vi "Avs47Ave.vi"() -> ()   [LabVIEW 2012]
doc: "Application example"
uses:
  <vilib>/ptbypt/NI_PtbyPt.lvlib
panel:
  out "VISA RESOURCE":refnum<visa-resource-name>
  in  "FIXED/AUTOSCALE":bool=TRUE
  out "AUTOSCALE CHART":i32(graph)
  in  "OFFSET/SCALE ADJ.":bool=TRUE
  out "AL ERROR":bool
  out "PEAK-TO-PEAK":dbl format="%_3f"
  out "LAST READING  AS STRING":string="000.000 ohm"
  out "PP/STD RATIO":dbl format="%.1f"
  out "READING No.":i32=1
  out "turns":i32
  in  "SAMPLE LENGTH":i32=300
  in  "RE-START MEASUREMENT":bool
  out "AVERAGE":dbl format="%^_5e"
  out "STD":dbl format="%_3f"
  out "FIXED SCALE CHART":i32(graph)
  out "LABVIEW ERROR":errorcluster
  out "OVERRANGE":bool
  out "ADC READING":i32
  in  "stop":bool
  in  "DIGITAL REFERENCE":u16 max=20475 step=1
  in  "DISPLAY":u8(ring) items=["530A SET PT"=7, "530A HEAT I"=6, "530A HEAT V"=5, "EXC VOLT"=4, "REFERENCE"=3, "ADJ REF"=2, "DR"=1, "R"=0]
  in  "EXCITATION":u8(ring)=7 items=["3mV"=7, "1mV"=6, "300uV"=5, "100uV"=4, "30uV"=3, "10uV"=2, "3 uV"=1, "NO EXCITATION"=0]
  in  "RANGE":u8(ring)=3 items=["2 MOhms"=7, "200 kOhms"=6, "20 kOhms"=5, "2 kOhms"=4, "200 Ohms"=3, "20 Ohms"=2, "2 Ohms"=1, "NO RANGE"=0]
  in  "CHANNEL":u8(ring) items=["CH7"=7, "CH6"=6, "CH5"=5, "CH4"=4, "CH3"=3, "CH2"=2, "CH1"=1, "CH0"=0]
  in  "INPUT":u8(ring)=2 items=["CAL"=2, "MEAS"=1, "ZERO"=0]
  in  "REMOTE":u8(ring) items=["YES"=1, "NO"=0]
  # "AVS47AVE.VI  NOISE AND CALIBRATION TEST PROGRAM FOR AVS-47B"
  # "RV-ELEKTRONIIKKA OY\nPICOWATT"
  # "The following port has been opened for the\nVISA session."
  # "NOTE 1:  Following settings must be made before starting the program: Sample length, Manual/Autoscale, Offset/Scale adj.\nNOTE 2:  Check the port that your computer is using as the VISA resource for the USB-232 converter.  Load, modify and run \n                 \"CreateDefaultConfigurationCluster.vi\" if it indicated an incorrect VISA resource."
  # "This VI can be used for testing the AVS-47B both in remote and local modes. The main use is testing noise and adjusting scale factor for the seven\nexcitation ranges. The bridge configuration can be changed after the program has started. Recording data can be re-started when\nrunning. \n\n- LAST READING is the AVS-47B display,  shown as a string with resistance unit appended for convenient reading.\n- AVERAGE is the mean value of [sample length] readings in ohms. If sample length has not yet been reached, AVERAGE  is the mean of \n   readings taken so far.\n- STD is the standard deviation of [sample length] readings in ohms. If sample length has not yet been reached, STD is the standard deviation\n   of readings taken so far.\n- PP/STD ratio should be about 5 for random noise and a large number of samples. A number much less than 5 is probably due to\n  too few readings. A number much higher than 5 is probably due to external interference (spikes), or too few samples.  On high excitation\n   ranges, digital steps can produce too low or too high PP/STD ratios.\n- ADC reading should be viewed if the DISPLAY is not R or 1xdR.  Calibration of excitation ranges should be done  at middle scale \n(reading 10000). \n- OVERRANGE indicator is set, if the voltage entering the A/D converter exceeds 1.9999 Volts (the ADC reading is  0 during overload)\n- AL ERROR tells that syncronisation to the ADC fails because the AL signal never comes true. This can happen if a wrong port was \n   opened as the  VISA resource, or if the  connection between AVS-47B and the computer fails.\n- If FIXED SCALE is selected, choose either OFFSET OR SCALE for \"OFFSET/SCALE ADJ\".  This centers the scale around 0 or 10000. The\n   low and high limits of the amplitude axis are automatically determined on the basis of the selected excitation range."
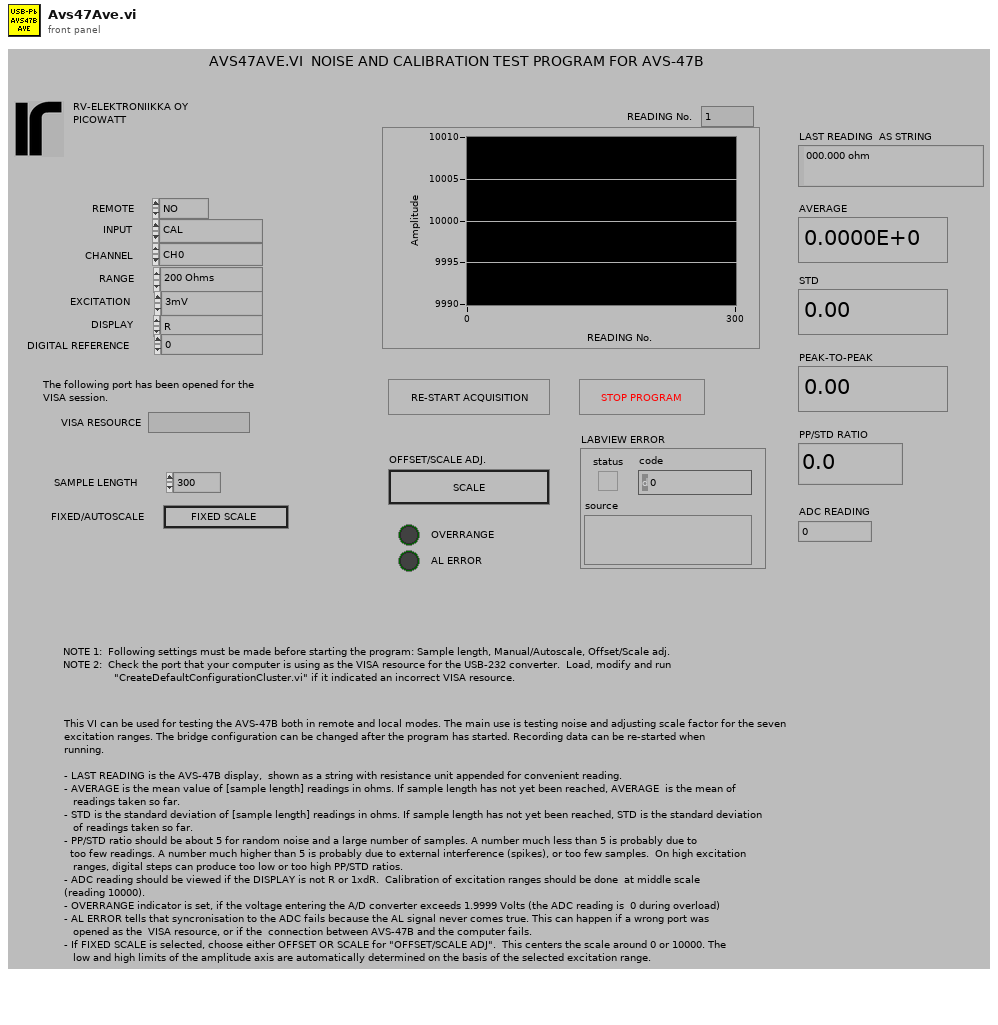
[diagram p1: front panel]
types:
  T1 = cluster{"VISA RESOURCE":refnum<visa-resource-name>, "PICOBUS ADDRESS":u8, "DISABLE AL":u8, "REMOTE":u8, "INPUT":u8, "CHANNEL":u8, "RANGE":u8, "EXCITATION":u8, "DISPLAY":u8, "DIGITAL REFERENCE":u16, "SET POINT":dbl, "PROP GAIN":u8, "INTG":u8, "DERIV":u8, "POWER BIAS":u8, "POWER RANGE":u8, "INFO STRING":string, "HEATER RESISTANCE":dbl, "INTERVAL":u8, " SENSOR dR/dT":u8}
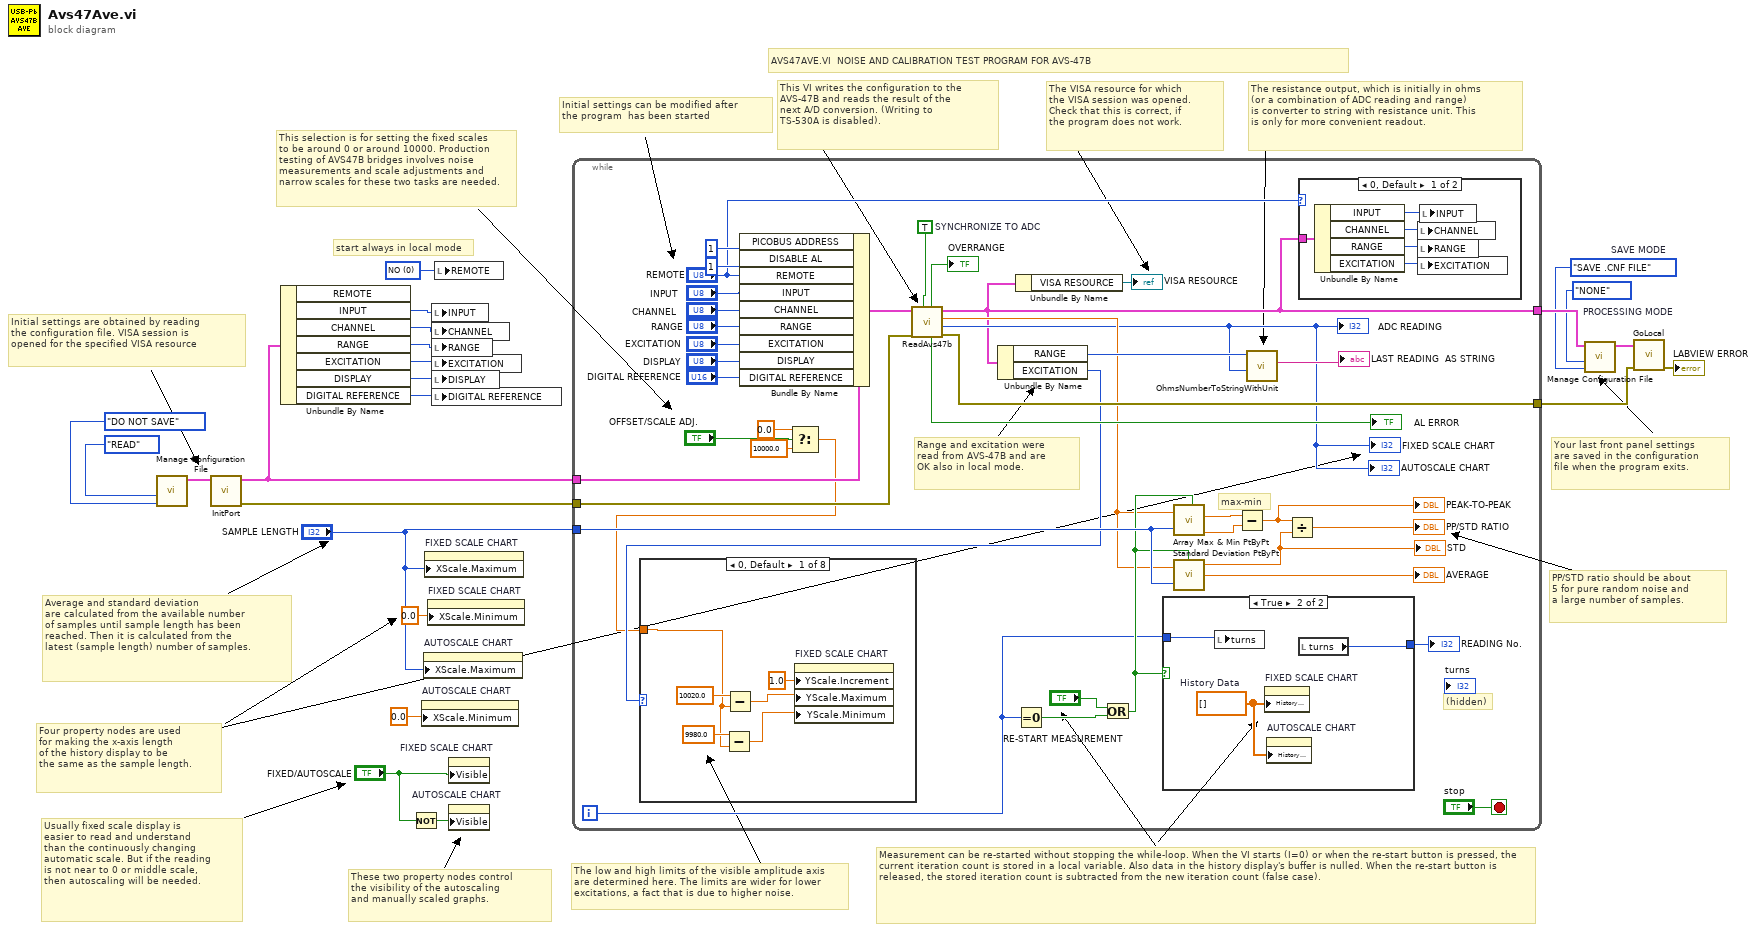
[diagram p0: block diagram]
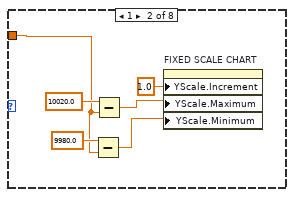
[diagram p3: hidden frame]
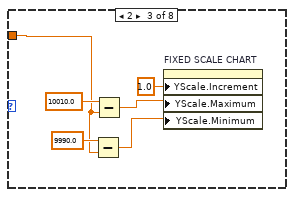
[diagram p4: hidden frame]
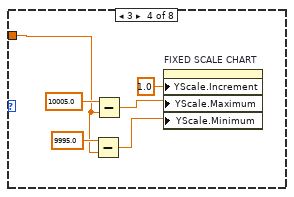
[diagram p5: hidden frame]
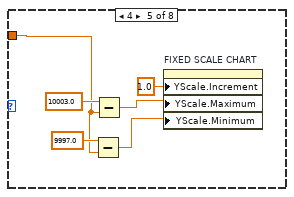
[diagram p6: hidden frame]
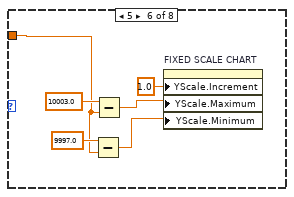
[diagram p7: hidden frame]
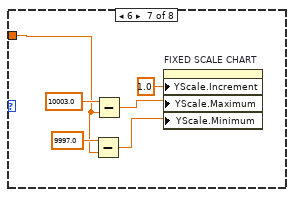
[diagram p8: hidden frame]
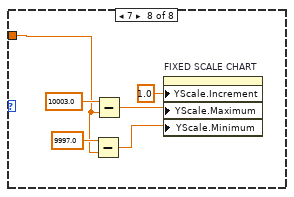
[diagram p9: hidden frame]
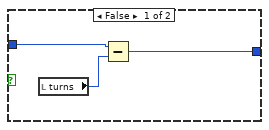
[diagram p10: hidden frame]
diagram:
  w7 = enum16{"NONE", "READ", "CREATE"}."NONE"  # PROCESSING MODE
  w6 = enum16{"DO NOT SAVE", "SAVE .CNF FILE"}."SAVE .CNF FILE"  # SAVE MODE
  w11 = u8 0 items=["YES"=1, "NO"=0] ("REMOTE")
  # "start always in local mode"
  # "The low and high limits of the visible amplitude axis\nare determined here. The limits are wider for lower\nexcitations, a fact that is due to higher noise."
  # "This selection is for setting the fixed scales\nto be around 0 or around 10000. Production\ntesting of AVS47B bridges involves noise\nmeasurements and scale adjustments and\nnarrow scales for these two tasks are needed."
  # "Measurement can be re-started without stopping the while-loop. When the VI starts (I=0) or when the re-start button is pressed, the current iteration count is stored in a local variable. Also data in the history display's buffer is nulled. When the re-start button is released, the stored iteration count is subtracted from the new iteration count (false case)."
  # "PP/STD ratio should be about\n5 for pure random noise and\na large number of samples."
  # "Your last front panel settings\nare saved in the configuration\nfile when the program exits."
  # "The resistance output, which is initially in ohms\n(or a combination of ADC reading and range)\nis converter to string with resistance unit. This\nis only for more convenient readout."
  # "The VISA resource for which\nthe VISA session was opened.\nCheck that this is correct, if\nthe program does not work."
  # "This VI writes the configuration to the\nAVS-47B and reads the result of the \nnext A/D conversion. (Writing to \nTS-530A is disabled)."
  # "Initial settings can be modified after\nthe program  has been started"
  # "These two property nodes control\nthe visibility of the autoscaling\nand manually scaled graphs."
  # "Usually fixed scale display is\neasier to read and understand\nthan the continuously changing\nautomatic scale. But if the reading\nis not near to 0 or middle scale,\nthen autoscaling will be needed."
  # "Four property nodes are used\nfor making the x-axis length\nof the history display to be \nthe same as the sample length."
  # "Average and standard deviation\nare calculated from the available number\nof samples until sample length has been \nreached. Then it is calculated from the \nlatest (sample length) number of samples."
  # "Initial settings are obtained by reading\nthe configuration file. VISA session is\nopened for the specified VISA resource"
  # "AVS47AVE.VI  NOISE AND CALIBRATION TEST PROGRAM FOR AVS-47B"
  n1 = call "Manage Configuration File.vi"("SAVE MODE"=enum16{"DO NOT SAVE", "SAVE .CNF FILE"}."DO NOT SAVE", "PROCESSING MODE"=enum16{"NONE", "READ", "CREATE"}."READ") -> ("CONFIGURATION CLUSTER OUT"=w5:T1)  [unwired: 9 in]
  n2 = call "InitPort.vi"("CONFIGURATION CLUSTER"=w5) -> ("LV ERROR OUT"=w1:errorcluster, "UNMODIFIED CONFIGURATION CLUSTER"=w2:T1)  [unwired: 6 in, 1 out]
  n3 = Unbundle By Name(w2) -> ("INPUT"=w17:u8, "CHANNEL"=w16:u8, "RANGE"=w15:u8, "EXCITATION"=w14:u8, "DISPLAY"=w13:u8, "DIGITAL REFERENCE"=w12:u16)  [unwired: 1 out]
  n4 = Not(x="FIXED/AUTOSCALE") -> (.not. x?=w20:bool)
  n5 = property on="AUTOSCALE CHART" class="WFChart (strict)"("XScale.Minimum"=0.0 ("X Scale.Range:Minimum")) -> ()  [unwired: 2 in, 2 out]
  n6 = property on="AUTOSCALE CHART" class="WFChart (strict)"("XScale.Maximum"="SAMPLE LENGTH") -> ()  [unwired: 2 in, 2 out]
  n7 = property on="FIXED SCALE CHART" class="WFChart (strict)"("XScale.Maximum"="SAMPLE LENGTH") -> ()  [unwired: 2 in, 2 out]
  n8 = property on="FIXED SCALE CHART" class="WFChart (strict)"("XScale.Minimum"=0.0 ("X Scale.Range:Minimum")) -> ()  [unwired: 2 in, 2 out]
  n9 = local write "INPUT"(w17) -> ()
  n10 = local write "CHANNEL"(w16) -> ()
  n11 = local write "RANGE"(w15) -> ()
  n12 = local write "EXCITATION"(w14) -> ()
  n13 = local write "DISPLAY"(w13) -> ()
  n14 = local write "DIGITAL REFERENCE"(w12) -> ()
  n15 = local write "REMOTE"(w11) -> ()
  n16 = property on="FIXED SCALE CHART" class="WFChart (strict)"("Visible"="FIXED/AUTOSCALE") -> ()  [unwired: 2 in, 2 out]
  n17 = property on="AUTOSCALE CHART" class="WFChart (strict)"("Visible"=w20) -> ()  [unwired: 2 in, 2 out]
  n18 = while {
    tunnel: w2 -> [w63]
    tunnel: w1 -> [w32]
    tunnel: "SAMPLE LENGTH" -> [w53]
    tunnel: [w25] -> w10
    tunnel: [w52] -> w9
    i -> [w34]
    stop <- "stop" stop-if-true
    w37 = TRUE  # SYNCHRONIZE TO ADC
    # "max-min"
    # "Range and excitation were\nread from AVS-47B and are\nOK also in local mode."
    # "(hidden)"
    n19 = Bundle By Name(cluster=w63, "PICOBUS ADDRESS"=u8 1, "DISABLE AL"=u8 1 ("PICOBUS ADDRESS"), "REMOTE"="REMOTE", "INPUT"="INPUT", "CHANNEL"="CHANNEL", "RANGE"="RANGE", "EXCITATION"="EXCITATION", "DISPLAY"="DISPLAY", "DIGITAL REFERENCE"="DIGITAL REFERENCE") -> (w54:T1)
    n20 = Select(t=0.0, s="OFFSET/SCALE ADJ.", f=10000.0) -> (s? t:f=w28:dbl)
    n21 = call "ReadAvs47b.vi"("SYNCHRONISE TO ADC"=w37, "LV ERROR IN"=w32, "CONFIGURATION CLUSTER"=w54) -> ("LV ERROR OUT"=w52:errorcluster, "ADC"=w27:i32, "RESISTANCE (OHMS)"=w36:sgl, "MODIFIED CONFIGURATION CLUSTER"=w25:T1, "WAITING FOR AL"=→"AL ERROR":bool, "ADC OVERRANGE"=→"OVERRANGE":bool)  [unwired: 3 in]
    "ADC READING" <- w27
    "FIXED SCALE CHART" <- w27
    "AUTOSCALE CHART" <- w27
    n22 = Unbundle By Name(w25) -> ("RANGE"=w38:u8, "EXCITATION"=w33:u8)
    n23 = case shown="0, Default" w33 {
      tunnel: w28 -> [w69 w75 w81 w87 w93 w99 w105 w111]
      frame 0, Default {
        n24 = Subtract(x=9980.0 ("Y Scale.Range:Increment"), y=w69) -> (x-y=w70:dbl)
        n25 = Subtract(x=10020.0 ("Y Scale.Range:Increment"), y=w69) -> (x-y=w72:dbl)
        n26 = property on="FIXED SCALE CHART" class="WFChart (strict)"("YScale.Increment"=1.0 ("Y Scale.Range:Increment"), "YScale.Maximum"=w72, "YScale.Minimum"=w70) -> ()  [unwired: 2 in, 2 out]
      }
      frame 1 {
        n27 = Subtract(x=9980.0 ("Y Scale.Range:Increment"), y=w75) -> (x-y=w76:dbl)
        n28 = Subtract(x=10020.0 ("Y Scale.Range:Increment"), y=w75) -> (x-y=w78:dbl)
        n29 = property on="FIXED SCALE CHART" class="WFChart (strict)"("YScale.Increment"=1.0 ("Y Scale.Range:Increment"), "YScale.Maximum"=w78, "YScale.Minimum"=w76) -> ()  [unwired: 2 in, 2 out]
      }
      frame 2 {
        n30 = Subtract(x=9990.0 ("Y Scale.Range:Increment"), y=w81) -> (x-y=w82:dbl)
        n31 = Subtract(x=10010.0 ("Y Scale.Range:Increment"), y=w81) -> (x-y=w84:dbl)
        n32 = property on="FIXED SCALE CHART" class="WFChart (strict)"("YScale.Increment"=1.0 ("Y Scale.Range:Increment"), "YScale.Maximum"=w84, "YScale.Minimum"=w82) -> ()  [unwired: 2 in, 2 out]
      }
      frame 3 {
        n33 = Subtract(x=9995.0 ("Y Scale.Range:Increment"), y=w87) -> (x-y=w88:dbl)
        n34 = Subtract(x=10005.0 ("Y Scale.Range:Increment"), y=w87) -> (x-y=w90:dbl)
        n35 = property on="FIXED SCALE CHART" class="WFChart (strict)"("YScale.Increment"=1.0 ("Y Scale.Range:Increment"), "YScale.Maximum"=w90, "YScale.Minimum"=w88) -> ()  [unwired: 2 in, 2 out]
      }
      frame 4 {
        n36 = Subtract(x=9997.0 ("Y Scale.Range:Increment"), y=w93) -> (x-y=w94:dbl)
        n37 = Subtract(x=10003.0 ("Y Scale.Range:Increment"), y=w93) -> (x-y=w96:dbl)
        n38 = property on="FIXED SCALE CHART" class="WFChart (strict)"("YScale.Increment"=1.0 ("Y Scale.Range:Increment"), "YScale.Maximum"=w96, "YScale.Minimum"=w94) -> ()  [unwired: 2 in, 2 out]
      }
      frame 5 {
        n39 = Subtract(x=9997.0 ("Y Scale.Range:Increment"), y=w99) -> (x-y=w100:dbl)
        n40 = Subtract(x=10003.0 ("Y Scale.Range:Increment"), y=w99) -> (x-y=w102:dbl)
        n41 = property on="FIXED SCALE CHART" class="WFChart (strict)"("YScale.Increment"=1.0 ("Y Scale.Range:Increment"), "YScale.Maximum"=w102, "YScale.Minimum"=w100) -> ()  [unwired: 2 in, 2 out]
      }
      frame 6 {
        n42 = Subtract(x=9997.0 ("Y Scale.Range:Increment"), y=w105) -> (x-y=w106:dbl)
        n43 = Subtract(x=10003.0 ("Y Scale.Range:Increment"), y=w105) -> (x-y=w108:dbl)
        n44 = property on="FIXED SCALE CHART" class="WFChart (strict)"("YScale.Increment"=1.0 ("Y Scale.Range:Increment"), "YScale.Maximum"=w108, "YScale.Minimum"=w106) -> ()  [unwired: 2 in, 2 out]
      }
      frame 7 {
        n45 = Subtract(x=9997.0 ("Y Scale.Range:Increment"), y=w111) -> (x-y=w112:dbl)
        n46 = Subtract(x=10003.0 ("Y Scale.Range:Increment"), y=w111) -> (x-y=w114:dbl)
        n47 = property on="FIXED SCALE CHART" class="WFChart (strict)"("YScale.Increment"=1.0 ("Y Scale.Range:Increment"), "YScale.Maximum"=w114, "YScale.Minimum"=w112) -> ()  [unwired: 2 in, 2 out]
      }
    }
    n48 = Unbundle By Name(w25) -> ("VISA RESOURCE"=→"VISA RESOURCE":refnum<visa-resource-name>)
    n49 = Equal To 0?(x=w34) -> (x = 0?=w47:bool)
    n50 = Or(x="RE-START MEASUREMENT", y=w47) -> (x .or. y?=w45:bool)
    n51 = case shown="True" w45 {
      tunnel: w34 -> [w119 w122]
      tunnel: [w117 w121] -> w50
      frame False {
        n52 = local read "turns"() -> (w118:i32)
        n53 = Subtract(x=w119, y=w118) -> (x-y=w117:i32)
      }
      frame True {
        w120 = sgl[] []  # History Data
        n54 = local write "turns"(w122) -> ()
        n55 = property on="FIXED SCALE CHART" class="WFChart (strict)"("History Data"=w120) -> ()  [unwired: 2 in, 2 out]
        n56 = property on="AUTOSCALE CHART" class="WFChart (strict)"("History Data"=w120) -> ()  [unwired: 2 in, 2 out]
        n57 = local read "turns"() -> (w121:i32)
      }
    }
    "READING No." <- w50
    n58 = call <vilib>:"Array Max & Min PtByPt.vi"("input data point"=w36, "sample length"=w53, "initialize"=w45) -> ("max value"=w49:dbl, "min value"=w48:dbl)  [unwired: 3 out]
    n59 = call <vilib>:"Standard Deviation PtByPt.vi"("x"=w36, "sample length"=w53, "initialize"=w45) -> ("standard deviation"=w44:dbl, "mean"=→"AVERAGE":dbl)  [unwired: 1 out]
    "STD" <- w44
    n60 = Subtract(x=w49, y=w48) -> (x-y=w41:dbl)
    "PEAK-TO-PEAK" <- w41
    n61 = call "OhmsNumberToStringWithUnit.vi"("ADC READING"=w27, "RANGE"=w38) -> ("RESISTANCE STRING"=→"LAST READING  AS STRING":string)  [unwired: 9 in]
    n62 = Divide(x=w41, y=w44) -> (x/y=→"PP/STD RATIO":dbl)
    n63 = case shown="0, Default" "REMOTE" {
      tunnel: w25 -> [w68 _]
      frame 0, Default {
        n64 = Unbundle By Name(w68) -> ("INPUT"=w64:u8, "CHANNEL"=w67:u8, "RANGE"=w66:u8, "EXCITATION"=w65:u8)
        n65 = local write "CHANNEL"(w67) -> ()
        n66 = local write "RANGE"(w66) -> ()
        n67 = local write "EXCITATION"(w65) -> ()
        n68 = local write "INPUT"(w64) -> ()
      }
      frame 1 {
      }
    }
  }
  n69 = call "Manage Configuration File.vi"("SAVE MODE"=w6, "PROCESSING MODE"=w7, "CONFIGURATION CLUSTER"=w10) -> ("CONFIGURATION CLUSTER OUT"=w8:T1)  [unwired: 8 in]
  n70 = call "GoLocal.vi"("LV ERROR IN"=w9, "CONFIGURATION CLUSTER"=w8) -> ("LV ERROR OUT"=→"LABVIEW ERROR":errorcluster)  [unwired: 9 in]
